vi "Delete User Attribute.vi"(0 "iUser Configuration Manager DVR":refnum<data-value>, 5 "Username":string, 7 "Attribute Name":string, 11 "error in":errorcluster) -> (4 "dup iUser Configuration Manager DVR":refnum<data-value>, 6 "Found":bool, 15 "error out":errorcluster)   [LabVIEW 2017, in "User Configuration Manager.lvlib" / "By Ref.lvlib"]
doc: "Deletes the attrbute specifed by attribute name from the user specifiec by user name."
uses:
  <vilib>/gpm_packages/@cs/user-manager/Source/User Configuration Manager Ref/By Ref.lvlib
  <vilib>/gpm_packages/@cs/user-manager/Source/iUser Configuration Manager/iUser Configuration Manager.lvclass
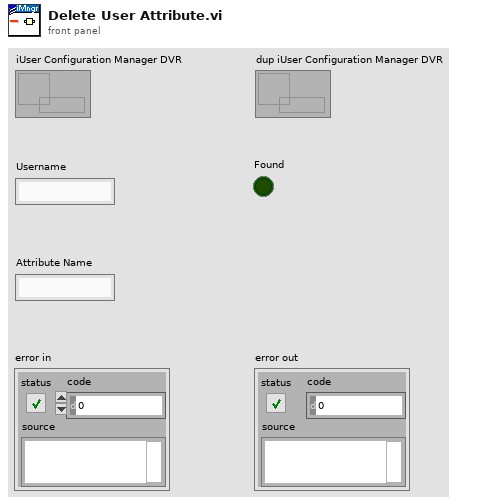
[diagram p1: front panel]
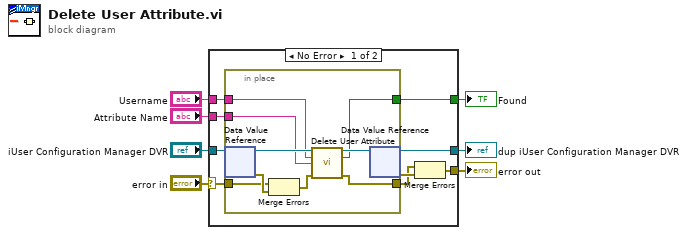
[diagram p0: block diagram]
diagram:
  n1 = case shown="No Error" "error in" {
    selector: "error in" -> [w14 w27]
    tunnel: "iUser Configuration Manager DVR" -> [w16 w26]
    tunnel: [w15 w27] -> w6
    tunnel: [w11 w26] -> w4
    tunnel: "Username" -> [w10 _]
    tunnel: "Attribute Name" -> [w9 _]
    tunnel: [w8 _] -> w1
    frame No Error {
      n2 = in-place "IPES" {
        in-place-border: [w20] -> w12
        in-place-border: w14 -> [w24]
        in-place-border: w10 -> [w19]
        in-place-border: w9 -> [w17]
        in-place-border: [w21] -> w8
        n3 = in-place-dvr #1(w16) -> (w23:refnum<class "iUser Configuration Manager.lvclass">, w25:errorcluster)
        n4 = Merge Errors(w24, w25) -> (w18:errorcluster)
        n5 = call-dynamic "Delete User Attribute.vi"("iUser Configuration Manager in"=w23, "Username"=w19, "Attribute Name"=w17, "error in (no error)"=w18) -> ("iUser Configuration Manager out"=w22:refnum<class "iUser Configuration Manager.lvclass">, "Found"=w21:bool, "error out"=w20:errorcluster)  [unwired: 9 in]
        n6 = in-place-dvr #1(w22) -> (w11:refnum<data-value>, w13:errorcluster)
      }
      n7 = Merge Errors(w12, w13) -> (w15:errorcluster)
    }
    frame Error {
    }
  }
  "error out" <- w6
  "dup iUser Configuration Manager DVR" <- w4
  "Found" <- w1
